vi "reset_method.vi"(5 "error in (no error)":errorcluster) -> (6 "Novo proteklo vrijeme":dbl, 7 "Novi vremenski trenutak":dbl, 8 "error out":errorcluster)   [LabVIEW 2023]
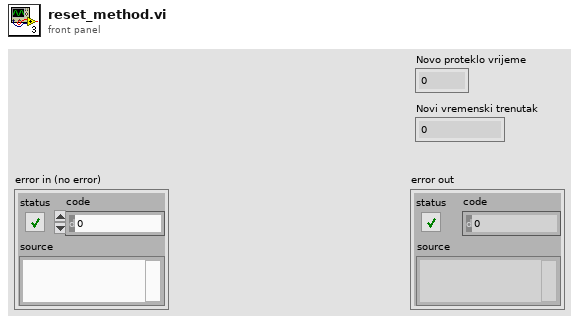
[diagram p1: front panel]
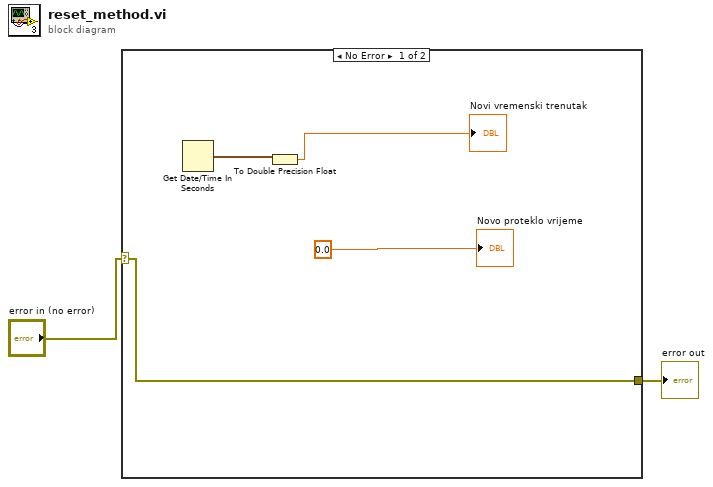
[diagram p0: block diagram]
diagram:
  n1 = case shown="No Error" "error in (no error)" {
    selector: "error in (no error)" -> [w6 w7]
    tunnel: [w6 w7] -> w1
    frame No Error {
      n2 = Get Date/Time In Seconds() -> (seconds since 1Jan1904=w4:timestamp)
      n3 = To Double Precision Float(number=w4) -> (double precision float=→"Novi vremenski trenutak":dbl)
      "Novo proteklo vrijeme" <- 0.0
    }
    frame Error {
    }
  }
  "error out" <- w1
